vi "RT_stagectrl_readIFO.vi"() -> ()   [LabVIEW 2019]
uses:
  <vilib>/Platform/TimedLoop/XDataNode/timing_clust.ctl
  <vilib>/Platform/TimedLoop/XDataNode/nitl_modes.ctl
  <vilib>/Platform/TimedLoop/XDataNode/wakeup.ctl
  <vilib>/Analysis/baseanly.llb/Mean (DBL).vi
  <vilib>/FPGAPlugInAG/myRIO-1900/niLvFpga_Open_myRIO-1900.vi
  <vilib>/rvi/interface/common/dynamic/niFpgaDynamicAddResources.vi
  <vilib>/Utility/error.llb/Error Cluster From Error Code.vi
  <vilib>/rvi/errors/niLvFpgaAdjustHostInterfaceError.vi
  <vilib>/FPGAPlugInAG/Dynamic/niLvFpga_Close_Dynamic.vi
  <vilib>/rvi/interface/nirviOpenFPGA/nirviOpenFPGA.xnode
  studentchallenge_FPGATarget_FPGA1RADC1WDAC2A_a-3TjVyjm4g.lvbitx
  <vilib>/rvi/interface/nirviReadWriteControl/nirviReadWriteControl.xnode
  <vilib>/platform/TimedLoop/XDataNode/XDataNode.xnode
  <vilib>/rvi/interface/nirviCloseFPGA/nirviCloseFPGA.xnode
  NiFpgaLv.dll
  <vilib>/rvi/interface/Simulation/niFpgaSimulationCallBeginRW.vi
  <vilib>/Platform/TimedLoop/XDataNode/XDNodeRunTimeDep.lvlib
  <vilib>/Analysis/NI_AALBase.lvlib
panel:
  out "Vrev":dbl=-3.5999999999999956
  out "Vfwd":dbl=0.2499999999999999
  out "Vd":dbl
  out "Vi":dbl=0.0203403515625
  out "Vp":dbl=6.7801171875
  out "late?":bool
  out "?":dynamicdata(graph)
  in  "Display signal plots comprimising IFO loop rate":bool
  out "Unit circle Lissajou":cluster{"X":dbl[], "Y":dbl[]}[](graph)
  out "?":dbl(graph)=0.0395625
  in  "IFO loop time (us)":i64=120
  in  "Stop":bool
  in  "P":dbl=1.0
  in  "I":dbl=0.003
  in  "D":dbl
  out "Control voltage":dbl=1.6749999999999978 format="%#_3f"
  out "Position (mm) 2":dbl=-2.725546875 format="%#_4f"
  out "late?":bool
  in  "Ramp ON":bool
  out "Mid-travel (mm)":dbl=4.0545703125 format="%#_3f"
  out "?":dynamicdata(graph)=[{"t0"=timestamp(2082849628.845535 s since 1904-01-01), "dt"=1.0, "Y"=[4.0545703125]}, {"t0"=timestamp(2082849628.845597 s since 1904-01-01), "dt"=1.0, "Y"=[-2.725546875]}]
  in  "Stage loop time (us)":i64=2000
  in  "Velocity (mm/s)":dbl=0.3 format="%#_3g"
  in  "Ramp Vpp (mm)":dbl=2.0 format="%#_13g"
  out "FWD limit flag":bool
  out "REV lim (mm)":dbl=-2.7246875 format="%#_5f"
  out "FWD lim (mm)":dbl=10.833828125 format="%#_5f"
  out "Voltage":dbl=3.5999999999999956
  out "REV limit flag":bool=TRUE
  out "Position (mm)":dbl(slide)=-2.7246875 scale=-10.0..10.0
  out "ENC0":i32=18
  out "Enc res (mm)":dbl=7.8125e-05
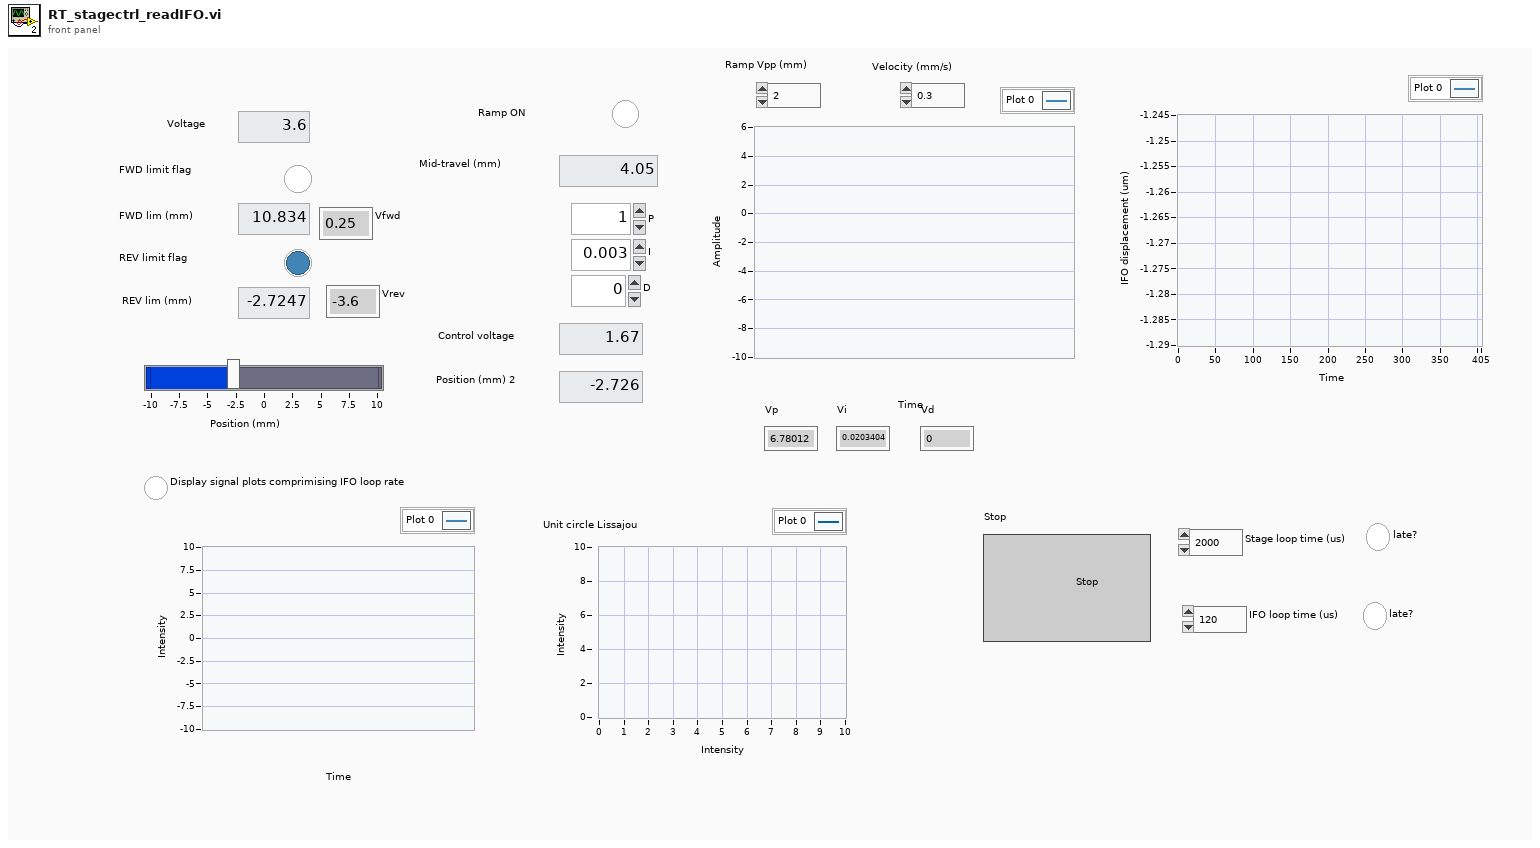
[diagram p1: front panel]
types:
  T1 = typedef "XDNodeRunTimeDep.lvlib/timing_clust.ctl" = cluster{"Expected End [f-1]":u64, "Actual End [f-1]":u64, "Finished Late? [f-1]":bool, "Expected End [i-1]":u64, "Actual End [i-1]":u64, "Finished Late? [i-1]":bool, "Expected Start [i]":u64, "Actual Start [i]":u64, "Expected Start [f]":u64, "Actual Start [f]":u64, "Source Name":string, "Structure Name":string, "Period":i64, "Deadline":i64, "Offset":i64, "Start":i64, "Priority":i32, "Timeout":i32, "Mode":T2, "Wakeup Reason":T3, "Error":errorcluster, "Source Type":string, "Secondary Source Type":string, "Global End Time":u64, "Global Start Time":u64, "Frame Duration":u64, "Iteration Duration":u64, "Assigned CPU":i32, "I/O Scan Engine Mode":u32}
  T2 = typedef "XDNodeRunTimeDep.lvlib/nitl_modes.ctl" = enum32{"No Change", "Process missed periods, maintain original phase", "Discard missed periods, maintain original phase", "Process missed periods, ignore original phase", "Discard missed periods, ignore original phase"}
  T3 = typedef "XDNodeRunTimeDep.lvlib/wakeup.ctl" = enum32{"Normal", "Aborted", "Asynchronous wakeup", "Timing source error", "Timed loop error", "Timeout"}
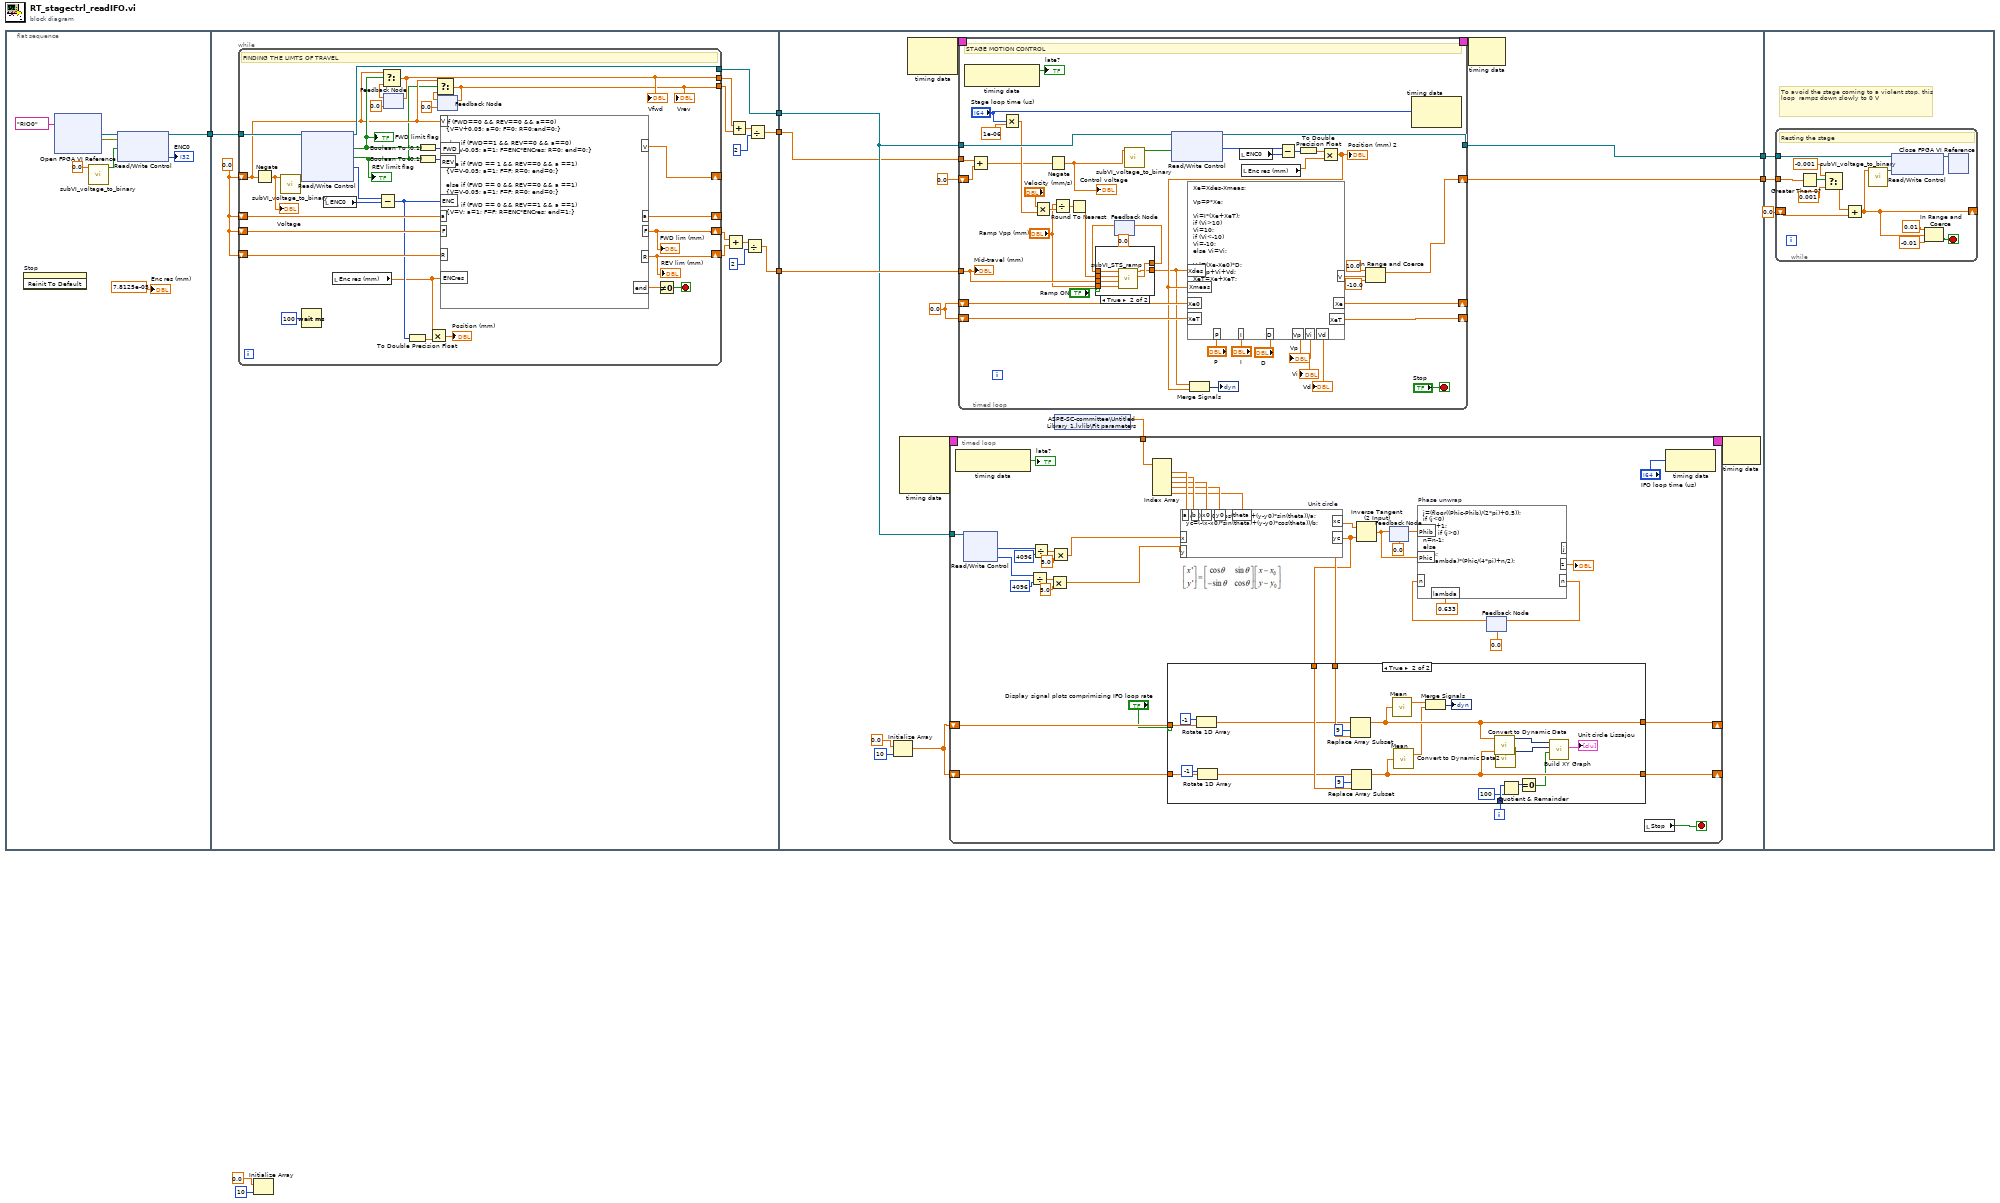
[diagram p0: block diagram]
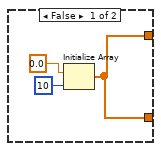
[diagram p2: hidden frame]
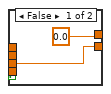
[diagram p3: hidden frame]
diagram:
  n1 = flat-sequence {
    tunnel: [w16] -> w8
    tunnel: w8 -> [w25]
    tunnel: [w22] -> w7
    tunnel: [w24] -> w6
    tunnel: [w17] -> w1
    tunnel: [w73] -> w5
    tunnel: w7 -> [w72]
    tunnel: w6 -> [w68]
    tunnel: [w71] -> w4
    tunnel: w1 -> [w62]
    tunnel: w5 -> [w205]
    tunnel: w4 -> [w204]
    frame #0 {
      n2 = invoke on="Stop" class="Bool (strict)" method="Reinit To Default"() -> ()  [unwired: 3 in, 3 out]
      n3 = xnode "Open FPGA VI Reference"("resource name"=tag "RIO0") -> ("FPGA VI Reference Out"=w9:refnum<k20>, "error out"=w14:errorcluster)  [unwired: 1 in]
      n4 = call "subVI_voltage_to_binary.vi"("voltage"=0.0) -> ("binary"=w12:bool[])  [unwired: 10 in]
      n5 = xnode "Read/Write Control"("FPGA VI Reference In"=w9, "error in"=w14, "DAC 1 write"=w12) -> ("FPGA VI Reference Out"=w16:refnum<k20>, "Encoder A"=→"ENC0":i32)  [unwired: 1 out]
      "Enc res (mm)" <- 7.8125e-05 ("y")
    }
    frame #1 {
      w23 = 0.0 ("V")
      n6 = while {
        shift-right: [w44] -> _
        shift-left: w23 -> [w33]
        shift-right: [w60] -> _
        shift-left: w23 -> [w59]
        shift-right: [w45] -> w27
        shift-left: w23 -> [w53]
        shift-right: [w46] -> w26
        shift-left: w23 -> [w52]
        tunnel: w25 -> [w50]
        tunnel: [w48] -> w24
        tunnel: [w31] -> w20
        tunnel: [w30] -> w19
        stop <- w55 stop-if-true
        # "FINDING THE LIMTS OF TRAVEL"
        n7 = Negate(x=w33) -> (-x=w39:dbl)
        "Voltage" <- w39
        n8 = call "subVI_voltage_to_binary.vi"("voltage"=w39) -> ("binary"=w51:bool[])  [unwired: 10 in]
        n9 = xnode "Read/Write Control"("FPGA VI Reference In"=w50, "DAC 1 write"=w51) -> ("FPGA VI Reference Out"=w48:refnum<k20>, "YFWD"=w38:bool, "YREV"=w32:bool, "Encoder A"=w54:i32)  [unwired: 1 in, 1 out]
        "FWD limit flag" <- w38
        "REV limit flag" <- w32
        n10 = Wait (ms)(milliseconds to wait=u32 100) -> ()  [unwired: 1 out]
        n11 = local read "ENC0"() -> (w49:i32)
        n12 = local read "Enc res (mm)"() -> (w41:dbl)
        n13 = Subtract(x=w54, y=w49) -> (x-y=w43:i32)
        n14 = feedback #1(0.0 ("V")) -> (w37:dbl)
        n15 = Select(t=w33, s=w38, f=w37) -> (s? t:f=w31:dbl)
        "Vfwd" <- w31
        n16 = feedback-in #1(w31) -> ()
        n17 = To Double Precision Float(number=w43) -> (double precision float=w40:dbl)
        n18 = Boolean To (0,1)(Boolean=w38) -> (0, 1=w58:i16)
        n19 = Boolean To (0,1)(Boolean=w32) -> (0, 1=w57:i16)
        n20 = Multiply(x=w41, y=w40) -> (x*y=→"Position (mm)":dbl)
        n21 = feedback #2(0.0 ("V")) -> (w35:dbl)
        n22 = Select(t=w33, s=w32, f=w35) -> (s? t:f=w30:dbl)
        "Vrev" <- w30
        n23 = feedback-in #2(w30) -> ()
        n24 = formula code="if (FWD==0 && REV==0 && a==0)\n{V=V+0.05; a=0; F=0; R=0;end=0;}\n\nelse if (FWD==1 && REV==0 && a==0)\n{V=V-0.05; a=1; F=ENC*ENCres; R=0; end=0;}\n\nelse if (FWD == 1 && REV==0 && a ==1)\n{V=V-0.05; a=1; F=F; R=0; end=0;}\n\nelse if (FWD == 0 && REV==0 && a ==1)\n{V=V-0.05; a=1; F=F; R=0; end=0;}\n\nelse if (FWD == 0 && REV==1 && a ==1)\n{V=V; a=1; F=F; R=ENC*ENCres; end=1;}"("FWD"=w58, "REV"=w57, "a"=w59, "ENC"=w43, "F"=w53, "R"=w52, "V"=w33, "ENCres"=w41) -> ("V"=w44:dbl, "a"=w60:dbl, "end"=w56:dbl, "F"=w45:dbl, "R"=w46:dbl)
        "REV lim (mm)" <- w46
        "FWD lim (mm)" <- w45
        n25 = Not Equal To 0?(x=w56) -> (x != 0?=w55:bool)
      }
      n26 = Add(x=w27, y=w26) -> (x+y=w29:dbl)
      n27 = Add(x=w20, y=w19) -> (x+y=w18:dbl)
      n28 = Divide(x=w29, y=2) -> (x/y=w22:dbl)
      n29 = Divide(x=w18, y=2) -> (x/y=w17:dbl)
    }
    frame #2 {
      w64 = 0.0 ("Xe")
      n30 = Initialize Array(0.0 ("element"), 10 ("dimension size")) -> (w65:dbl[])
      n31 = node-c288() -> (w70:T1)  [unwired: 4 in]
      n32 = node-c288() -> (w75:T1)  [unwired: 2 in]
      n33 = timed-loop {
        timing: w75 -> [_]
        timing-out: [_] -> w74
        tunnel: [w183] -> w73
        tunnel: w72 -> [w153]
        shift-right: [w168] -> w71
        shift-left: 0.0 ("upper limit") -> [w147]
        tunnel: w68 -> [w181]
        shift-right: [w176] -> _
        shift-left: w64 -> [w175]
        shift-right: [w174] -> _
        shift-left: w64 -> [w173]
        tunnel: w62 -> [w146]
        stop <- "Stop" stop-if-true
        # "STAGE MOTION CONTROL"
        n34 = node-c288() -> (→"late?":bool)  [unwired: 1 in]
        n35 = Add(x=w146, y=w147) -> (x+y=w144:dbl)
        n36 = Multiply(x="Stage loop time (us)", y=1e-06) -> (x*y=w161:dbl)
        n37 = Multiply(x="Velocity (mm/s)", y=w161) -> (x*y=w164:dbl)
        n38 = Negate(x=w144) -> (-x=w145:dbl)
        "Control voltage" <- w145
        n39 = Divide(x="Ramp Vpp (mm)", y=w164) -> (x/y=w159:dbl)
        n40 = Round To Nearest(number=w159) -> (nearest integer value=w154:dbl)
        n41 = feedback #3(0.0 ("n1")) -> (w156:dbl)
        n42 = case shown="True" "Ramp ON" {
          tunnel: w156 -> [_ w195]
          tunnel: [0.0 ("n1") w194] -> w155
          tunnel: w154 -> [_ w193]
          tunnel: w153 -> [w189 w192]
          tunnel: [w189 w191] -> w151
          tunnel: "Ramp Vpp (mm)" -> [_ w190]
          frame False {
          }
          frame True {
            n43 = call "subVI_STS_ramp.vi"("Ramp Vpp"=w190, "Ramp offset"=w192, "Ramp datapoints"=w193, "n"=w195) -> ("n1"=w194:dbl, "Ramp out"=w191:dbl)  [unwired: 6 in]
          }
        }
        n44 = feedback-in #3(w155) -> ()
        n45 = call "subVI_voltage_to_binary.vi"("voltage"=w145) -> ("binary"=w184:bool[])  [unwired: 10 in]
        n46 = xnode "Read/Write Control"("FPGA VI Reference In"=w181, "DAC 1 write"=w184) -> ("FPGA VI Reference Out"=w183:refnum<k20>, "Encoder A"=w185:i32)  [unwired: 1 in, 1 out]
        n47 = local read "ENC0"() -> (w182:i32)
        n48 = local read "Enc res (mm)"() -> (w165:dbl)
        n49 = Subtract(x=w185, y=w182) -> (x-y=w186:i32)
        n50 = To Double Precision Float(number=w186) -> (double precision float=w187:dbl)
        n51 = Multiply(x=w187, y=w165) -> (x*y=w166:dbl)
        "Position (mm) 2" <- w166
        n52 = formula code="Xe=Xdes-Xmeas;\n\nVp=P*Xe;\n\nVi=I*(Xe+XeT);\nif (Vi>10)\nVi=10;\nif (Vi<-10)\nVi=-10;\nelse Vi=Vi;\n\nVd=(Xe-Xe0)*D;\nV=Vp+Vi+Vd;\nXeT=Xe+XeT;"("Xdes"=w151, "Xmeas"=w166, "Xe0"=w175, "XeT"=w173, "P"="P", "I"="I", "D"="D") -> ("Xe"=w176:dbl, "V"=w177:dbl, "XeT"=w174:dbl, "Vp"=→"Vp":dbl, "Vi"=→"Vi":dbl, "Vd"=→"Vd":dbl)
        n53 = Merge Signals(w151, w166) -> (→"?":dynamicdata)
        n54 = In Range and Coerce(upper limit=10.0, x=w177, lower limit=-10.0) -> (coerced(x)=w168:dbl)  [unwired: 1 out]
        n55 = node-c288("Stage loop time (us)") -> ()  [unwired: 1 in, 1 out]
        "Mid-travel (mm)" <- w153
      }
      n56 = shared-variable "ASPE-SC-committee\\Untitled Library 1.lvlib\\Fit parameters"() -> (w61:dbl[])  [unwired: 1 in, 1 out]
      n57 = timed-loop {
        shift-right: [w109] -> _
        shift-left: w65 -> [w111]
        shift-right: [w108] -> _
        shift-left: w65 -> [w110]
        timing: w70 -> [_]
        timing-out: [_] -> w69
        tunnel: w68 -> [w102]
        tunnel: w61 -> [w80]
        i -> [w107]
        stop <- w77 stop-if-true
        n58 = node-c288() -> (→"late?":bool)  [unwired: 1 in]
        n59 = xnode "Read/Write Control"("FPGA VI Reference In"=w102) -> ("PD1"=w101:u16, "PD2"=w94:u16)  [unwired: 1 in, 2 out]
        n60 = Divide(x=w94, y=u16 4096) -> (x/y=w96:dbl)
        n61 = Divide(x=w101, y=u16 4096) -> (x/y=w99:dbl)
        n62 = Multiply(x=w96, y=5.0) -> (x*y=w92:dbl)
        n63 = Multiply(x=w99, y=5.0) -> (x*y=w97:dbl)
        n64 = Index Array(array=w80) -> (element #1=w91:dbl, element #2=w90:dbl, element #3=w89:dbl, element #4=w88:dbl, element #5=w87:dbl)  [unwired: 5 in]
        n65 = formula code="xc=((x-x0)*cos(theta)+(y-y0)*sin(theta))/a;\nyc=(-(x-x0)*sin(theta)+(y-y0)*cos(theta))/b;" "Unit circle"("a"=w91, "b"=w90, "x0"=w89, "y0"=w88, "theta"=w87, "x"=w97, "y"=w92) -> ("yc"=w105:dbl, "xc"=w106:dbl)
        n66 = case shown="True" "Display signal plots comprimising IFO loop rate" {
          tunnel: w111 -> [_ w136]
          tunnel: w110 -> [_ w135]
          tunnel: [w112 w134] -> w109
          tunnel: [w112 w133] -> w108
          tunnel: w107 -> [_ w132]
          tunnel: w106 -> [_ w131]
          tunnel: w105 -> [_ w130]
          frame False {
            n67 = Initialize Array(0.0 ("element"), 10 ("dimension size")) -> (w112:dbl[])
          }
          frame True {
            n68 = Rotate 1D Array(1:w136, 2:-1 ("n")) -> (0:w128:dbl[])
            n69 = Rotate 1D Array(1:w135, 2:-1 ("n")) -> (0:w125:dbl[])
            n70 = Replace Array Subset(array=w128, new element=w131, index=9) -> (w134:dbl[])
            n71 = Replace Array Subset(array=w125, new element=w130, index=9) -> (w133:dbl[])
            n72 = call-poly <vilib>:"Mean.vi"("X"=w134) -> ("mean"=w117:dbl)  [unwired: 1 out]
            n73 = call-poly <vilib>:"Mean.vi"("X"=w133) -> ("mean"=w116:dbl)  [unwired: 1 out]
            n74 = Merge Signals(w117, w116) -> (→"?":dynamicdata)
            n75 = call "Convert to Dynamic Data"("Array"=w134) -> ("Dynamic Data Type"=w123:dynamicdata)  [unwired: 3 in]
            n76 = call "Convert to Dynamic Data2"("Array"=w133) -> ("Dynamic Data Type"=w122:dynamicdata)  [unwired: 3 in]
            n77 = Quotient & Remainder(x=w132, y=100) -> (x-y*floor(x/y)=w119:i32)  [unwired: 1 out]
            n78 = Equal To 0?(x=w119) -> (x = 0?=w120:bool)
            n79 = call "Build XY Graph"("Reset"=w120, "Y Input"=w122, "X Input"=w123) -> ("XY Graph"=→"Unit circle Lissajou":cluster{"X":dbl[], "Y":dbl[]}[])  [unwired: 7 in, 1 out]
          }
        }
        n80 = Inverse Tangent (2 Input)(1:w105, 2:w106) -> (0:w83:dbl)
        n81 = feedback #4(0.0) -> (w84:dbl)
        n82 = feedback-in #4(w83) -> ()
        n83 = feedback #5(0.0 ("j")) -> (w85:dbl)
        n84 = formula code="j=(floor((Phic-Phib)/(2*pi)+0.5));\nif (j<0)\nn=n+1;\nelse if (j>0)\nn=n-1;\nelse\nn=n;\nz=(lambda)*(Phic/(4*pi)+n/2);" "Phase unwrap"("Phic"=w83, "Phib"=w84, "n"=w85, "lambda"=0.633 ("input variable")) -> ("n"=w82:dbl, "z"=→"?":dbl)  [unwired: 1 out]
        n85 = feedback-in #5(w82) -> ()
        n86 = local read "Stop"() -> (w77:bool)
        n87 = node-c288("IFO loop time (us)") -> ()  [unwired: 1 out]
      }
      n88 = node-c288(w74) -> ()  [unwired: 1 out]
      n89 = node-c288(w69) -> ()  [unwired: 1 out]
    }
    frame #3 {
      # "To avoid the stage coming to a violent stop, this loop  ramps down slowly to 0 V"
      n90 = while {
        tunnel: w205 -> [w216]
        tunnel: w204 -> [w207]
        shift-right: [w206] -> _
        shift-left: 0.0 -> [w211]
        stop <- w208 stop-if-true
        # "Resting the stage"
        n91 = Greater Than 0?(x=w207) -> (x > 0?=w215:bool)
        n92 = Select(t=-0.001, s=w215, f=0.001) -> (s? t:f=w212:dbl)
        n93 = Add(x=w212, y=w211) -> (x+y=w206:dbl)
        n94 = call "subVI_voltage_to_binary.vi"("voltage"=w206) -> ("binary"=w218:bool[])  [unwired: 10 in]
        n95 = xnode "Read/Write Control"("FPGA VI Reference In"=w216, "DAC 1 write"=w218) -> ("FPGA VI Reference Out"=w217:refnum<k20>)  [unwired: 1 in, 1 out]
        n96 = In Range and Coerce(upper limit=0.01, x=w206, lower limit=-0.01) -> (In Range?=w208:bool)  [unwired: 1 out]
        n97 = xnode "Close FPGA VI Reference"("FPGA VI Reference In"=w217) -> ()  [unwired: 1 in, 1 out]
      }
    }
  }
  n98 = Initialize Array(0.0 ("element"), 10 ("dimension size")) -> ()  [unwired: 1 out]
